vi "ge_GetGrpChans_1Grp.vi"(10 "Chassis Name":tag, 11 "GroupChansIn":refnum<class "Channel.lvclass">[](array[class])) -> (1 "Num of Chans":i32, 2 "Multi Rate Mods in Grp":T1, 3 "GroupChansOut":refnum<class "Channel.lvclass">[](array[class]), 4 "Chans w/ Modbus":i32[](array[numeric]), 5 "Chan Aliases":string[][](array[string]))   [LabVIEW 2011]
uses:
  Custom Ctrls Bld/ge_MultiRateMods.ctl
  Classes/Channel/Channel.lvclass
  Classes/Channel/Read Device.vi
  Classes/Channel/Read ChanName.vi
  Classes/Channel/Read Alias.vi
  Classes/Channel/Read ModbusAddr.vi
  Classes/Channel/Read ToModBus.vi
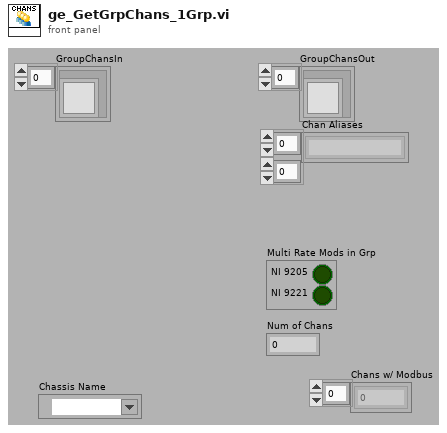
[diagram p1: front panel]
types:
  T1 = typedef "ge_MultiRateMods.ctl" = cluster{"NI 9205":bool, "NI 9221":bool}
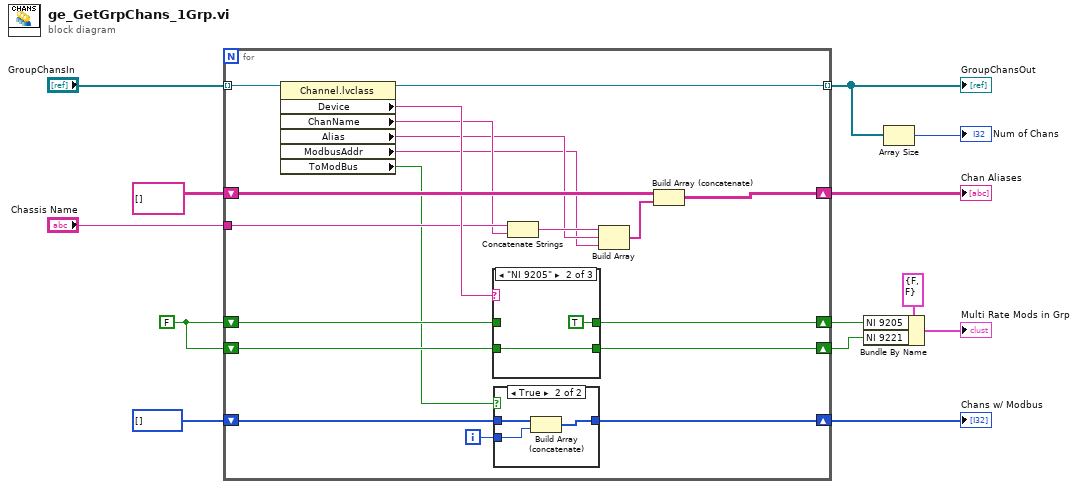
[diagram p0: block diagram]
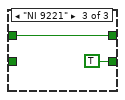
[diagram p4: hidden frame]
diagram:
  w12 = FALSE
  n1 = for {
    tunnel: "GroupChansIn" -> [w22] mode=indexing
    shift-right: [w30] -> w11
    shift-left: w12 -> [w32]
    shift-right: [w29] -> w10
    shift-left: w12 -> [w31]
    tunnel: "Chassis Name" -> [w19]
    tunnel: [w21] -> w4 mode=indexing
    shift-right: [w26] -> w5
    shift-left: i32[] [] -> [w28]
    shift-right: [w23] -> w2
    shift-left: string[][] [] -> [w25]
    i -> [w27]
    n2 = property class="Channel.lvclass"(reference=w22) -> (reference out=w21:refnum<class "Channel.lvclass">, "Device"=w20:string, "ChanName"=w18:string, "Alias"=w16:string, "ModbusAddr"=w15:string, "ToModBus"=w14:bool)  [unwired: 1 in, 1 out]
    n3 = case shown="\"NI 9205\"" w20 {
      tunnel: w32 -> [w38 _ w42]
      tunnel: w31 -> [w37 w39 _]
      tunnel: [w38 TRUE w42] -> w30
      tunnel: [w37 w39 TRUE] -> w29
      frame Default {
      }
      frame "NI 9205" {
      }
      frame "NI 9221" {
      }
    }
    n4 = case shown="True" w14 {
      tunnel: w28 -> [w33 w36]
      tunnel: w27 -> [_ w35]
      tunnel: [w33 w34] -> w26
      frame False {
      }
      frame True {
        n5 = Build Array (concatenate)(w36, w35) -> (w34:i32[])
      }
    }
    n6 = Concatenate Strings(w19, w18) -> (w17:string)
    n7 = Build Array(w17, w16, w15) -> (w24:string[])
    n8 = Build Array (concatenate)(w25, w24) -> (w23:string[][])
  }
  "Chans w/ Modbus" <- w5
  "GroupChansOut" <- w4
  "Chan Aliases" <- w2
  n9 = Bundle By Name(cluster=T1 {"NI 9205"=FALSE, "NI 9221"=FALSE} ("Multi Rate Mods in Grp"), "NI 9205"=w11, "NI 9221"=w10) -> (→"Multi Rate Mods in Grp":T1)
  n10 = Array Size(array=w4) -> (size(s)=→"Num of Chans":i32)
